vi "Add Async Methods Actor.vi"(8 "error in":errorcluster, 11 "Target Item":T1) -> (0 "error out":errorcluster)   [LabVIEW 2023, in "Add Async Methods Actor.lvlib"]
uses:
  Add Async Methods Actor.lvlib
  <resource>/Framework/Providers/API/mxLvNIIM.ctl
  Classes/Live Store/Live Store.lvclass
  Localized Strings.vi
  AFPP Shared/AFPP Shared.lvlib
  C:/Users/AndreaVaccaro(LSInst/Downloads/Projects/Async Methods Actor/Providers/AddAsyncMethodsActor/Classes/Actor Store/Actor Store.lvclass
  C:/Users/AndreaVaccaro(LSInst/Downloads/Projects/Async Methods Actor/Providers/AddAsyncMethodsActor/Classes/Live Store/Live Store.lvclass
panel:
  out "Path Display":string
  in  "Path":path caption="Save files to..."
  in  "Inherit from:":string(combo)
  in  "Cancel Button":bool
  in  "OK Button":bool
  in  "Name of Async Method Actor":string
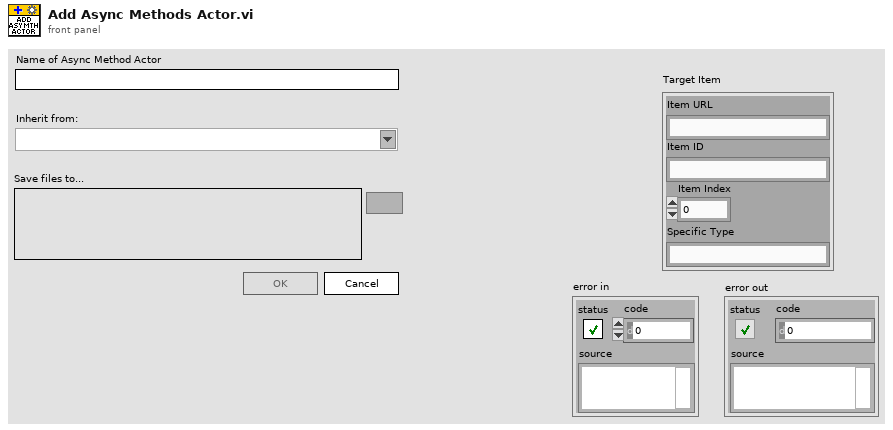
[diagram p1: front panel]
types:
  T1 = typedef "mxLvNIIM.ctl" = cluster{"Item URL":string, "Item ID":string, "Item Index":i32, "Specific Type":string}
  T2 = enum8{"Enabled", "Disabled", "Disabled and Grayed Out"}
  T3 = enum32{"Invalid", "Standard", "Closed", "Hidden", "Minimized", "Maximized"}
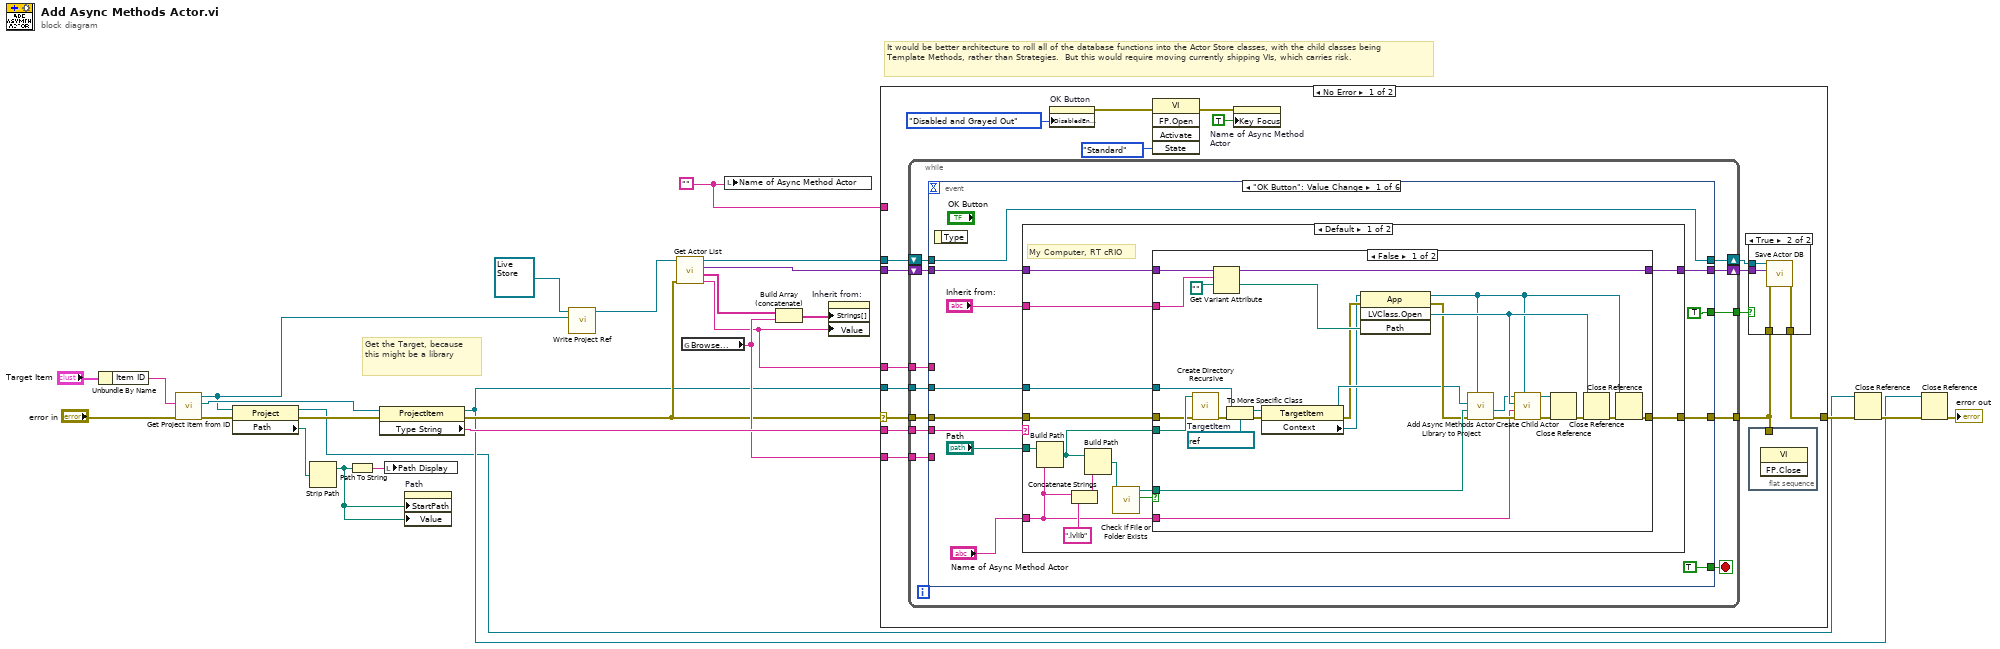
[diagram p0: block diagram]
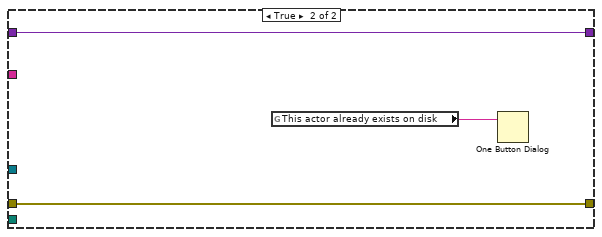
[diagram p2: hidden frame]
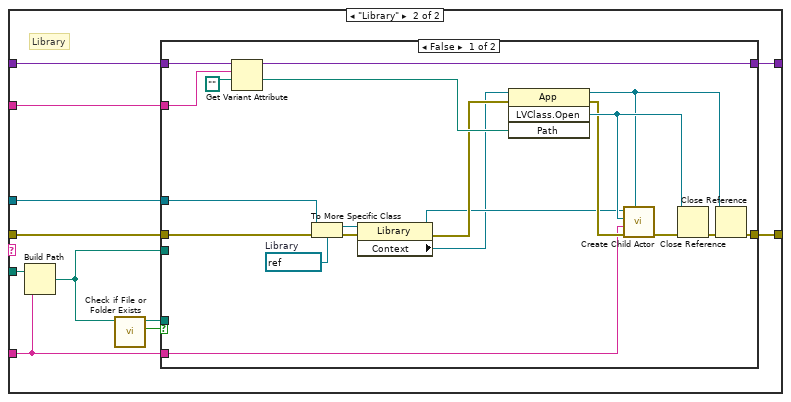
[diagram p3: hidden frame]
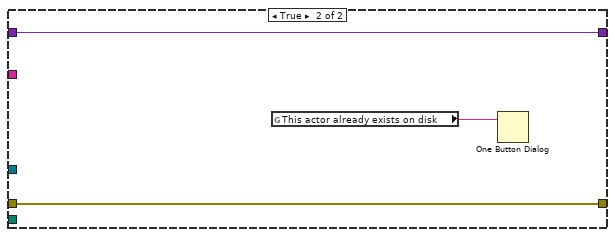
[diagram p4: hidden frame]
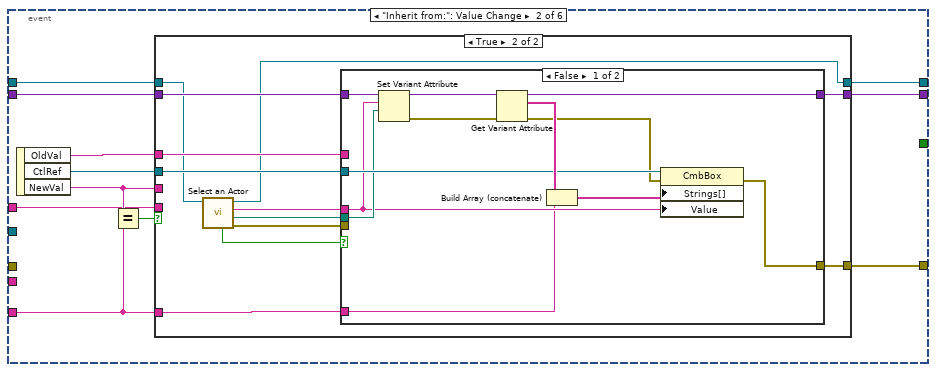
[diagram p5: hidden frame]
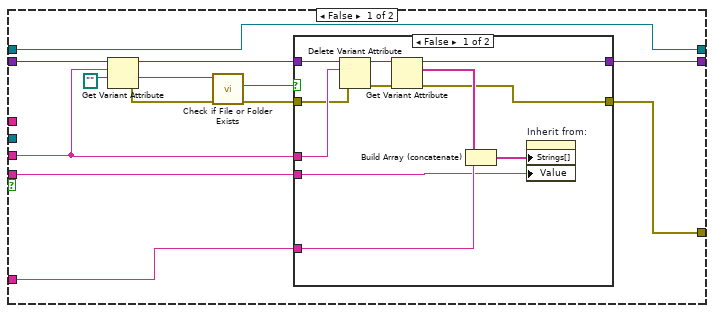
[diagram p6: hidden frame]
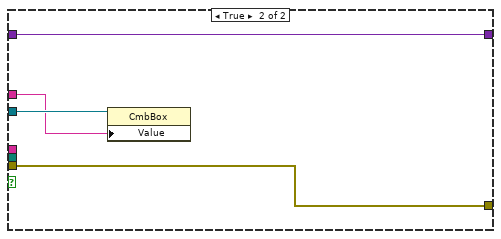
[diagram p8: hidden frame]
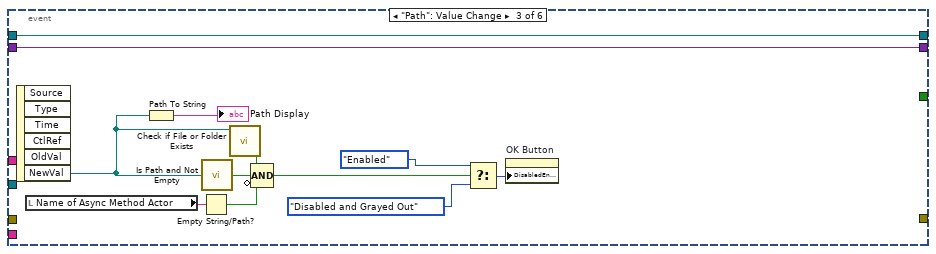
[diagram p9: hidden frame]
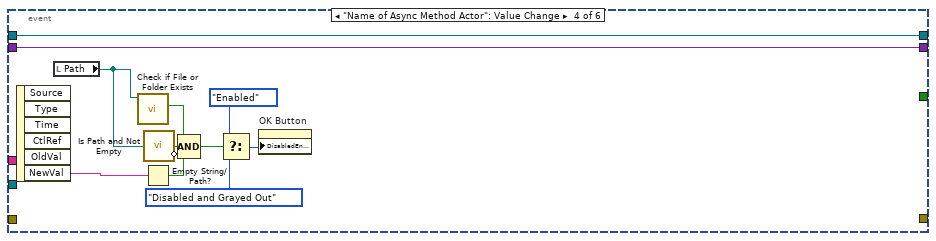
[diagram p10: hidden frame]
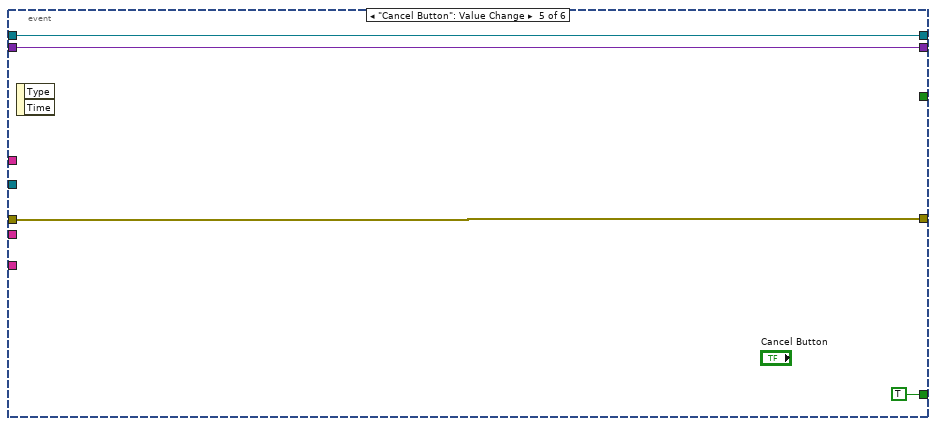
[diagram p11: hidden frame]
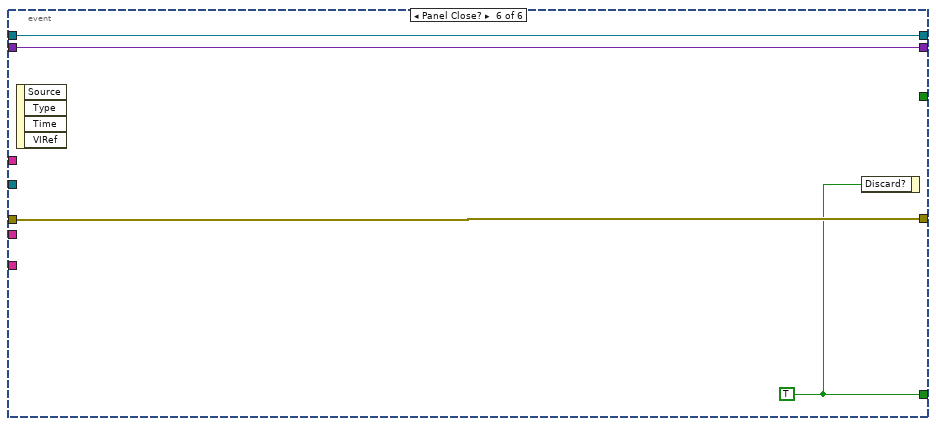
[diagram p12: hidden frame]
diagram:
  w10 = "" ("Name of Actor")
  # "Get the Target, because this might be a library"
  # "It would be better architecture to roll all of the database functions into the Actor Store classes, with the child classes being Template Methods, rather than Strategies.  But this would require moving currently shipping VIs, which carries risk."
  n1 = Unbundle By Name("Target Item") -> ("Item ID"=w7:string)
  n2 = call "Get Project Item from ID.vi"("error in (no error)"="error in", "Item ID"=w7) -> ("error out"=w4:errorcluster, "Project Item"=w3:refnum<vi>, "Project out"=w2:refnum<vi>)  [unwired: 7 in]
  n3 = property class="Project"(reference=w2, error in=w4) -> (reference out=w8:refnum<vi>, error out=w18:errorcluster, "Path"=w24:path)
  n4 = Strip Path(path=w24) -> (stripped path=w20:path)  [unwired: 1 out]
  n5 = Path To String(path=w20) -> (string=w21:string)
  n6 = property class="ProjectItem"(reference=w3, error in=w18) -> (reference out=w9:refnum<vi>, error out=w12:errorcluster, "Type String"=w23:string)
  n7 = local write "Path Display"(w21) -> ()
  n8 = property on="Path" class="Path"("StartPath"=w20, "Value"=w20) -> ()  [unwired: 2 in, 2 out]
  n9 = call-dynamic "Write Project Ref.vi"("Project Item"=w2, "Target Store in"=refnum<class "Live Store.lvclass"> refnum ("Add Async Methods Actor.lvlib:Live Store.lvclass")) -> ("Target Store out"=w17:refnum<class "Live Store.lvclass">)  [unwired: 9 in]
  n10 = call "Get Actor List.vi"("error in (no error)"=w12, "Actor Store"=w17) -> ("Actor Label"=w19:string, "Actors"=w15:string[], "Actor Paths"=w26:variant, "Actor Store"=w16:refnum<class "Live Store.lvclass">)  [unwired: 6 in]
  n11 = global read "Localized Strings.vi" "Browse..."() -> (w22:string)
  n12 = local write "Name of Async Method Actor"(w10) -> ()
  n13 = Build Array (concatenate)(w15, w22) -> (w25:string[])
  n14 = property on="Inherit from:" class="CmbBox"("Strings[]"=w25, "Value"=w19) -> ()  [unwired: 2 in, 2 out]
  n15 = case shown="No Error" w12 {
    selector: w12 -> [w43 w247]
    tunnel: [w37 w247] -> w13
    tunnel: w26 -> [w42 _]
    tunnel: w23 -> [w41 _]
    tunnel: w9 -> [w40 _]
    tunnel: w22 -> [w39 _]
    tunnel: w19 -> [w35 _]
    tunnel: w16 -> [w34 _]
    tunnel: w10 -> [_ _]
    frame No Error {
      n16 = while {
        tunnel: [w55] -> w31
        tunnel: w43 -> [w54]
        shift-right: [w51] -> w38
        shift-left: w42 -> [w52]
        tunnel: w41 -> [w50]
        tunnel: w40 -> [w49]
        tunnel: w39 -> [w48]
        tunnel: [w47] -> w36
        tunnel: w35 -> [w46]
        shift-right: [w44] -> w33
        shift-left: w34 -> [w45]
        stop <- w53 stop-if-true
        n17 = event shown="[0] \"OK Button\": Value Change" {
          selector: _ -> [_ _ _ _ _ _]
          dyn-events: _ -> [_ _ _ _ _ _]
          timeout: _ -> [_ _ _ _ _ _]
          tunnel: w54 -> [w61 _ _ _ w236 w241]
          tunnel: [w62 w156 _ _ w236 w241] -> w55
          tunnel: [TRUE _ _ _ TRUE w239] -> w53
          tunnel: w52 -> [w65 w155 w219 w226 w235 w240]
          tunnel: [w63 w154 w219 w226 w235 w240] -> w51
          tunnel: w50 -> [w60 _ _ _ _ _]
          tunnel: w49 -> [w59 _ _ _ _ _]
          tunnel: w48 -> [_ w150 _ _ _ _]
          tunnel: [TRUE _ _ _ _ _] -> w47
          tunnel: w46 -> [_ w149 _ _ _ _]
          tunnel: w45 -> [w56 w147 w211 w223 w234 w238]
          tunnel: [w56 w146 w211 w223 w234 w238] -> w44
          event "OK Button": Value Change {
            n18 = event-data() -> ()  [unwired: 1 in, 1 out]
            n19 = case shown="Default" w60 {
              tunnel: "Path" -> [w81 w122]
              tunnel: "Name of Async Method Actor" -> [w69 w113]
              tunnel: w65 -> [w80 w121]
              tunnel: "Inherit from:" -> [w79 w120]
              tunnel: [w78 w119] -> w63
              tunnel: [w75 w117] -> w62
              tunnel: w61 -> [w74 w116]
              tunnel: w59 -> [w72 w114]
              frame Default {
                # "My Computer, RT cRIO"
                n20 = Build Path(base path=w81, name or relative path=w69) -> (appended path=w77:path)
                n21 = Concatenate Strings(w69, ".lvlib" ("string")) -> (w70:string)
                n22 = Build Path(base path=w77, name or relative path=w70) -> (appended path=w68:path)
                n23 = call <vilib>:"Check if File or Folder Exists.vi"("path"=w68) -> ("file or folder exists?"=w73:bool, "dup path"=w76:path)  [unwired: 8 in, 1 out]
                n24 = case shown="False" w73 {
                  tunnel: w69 -> [w92 _]
                  tunnel: w80 -> [w107 w111]
                  tunnel: w79 -> [w106 _]
                  tunnel: [w105 w111] -> w78
                  tunnel: w77 -> [w91 _]
                  tunnel: w76 -> [w102 _]
                  tunnel: [w93 w110] -> w75
                  tunnel: w74 -> [w90 w110]
                  tunnel: w72 -> [w96 _]
                  frame False {
                    w101 = refnum<vi> refnum  # TargetItem
                    n25 = call <vilib>:"Create Directory Recursive.vi"("error in (no error)"=w90, "directory"=w91) -> ("error out"=w89:errorcluster)  [unwired: 3 in, 2 out]
                    n26 = Get Variant Attribute(Variant=w107, name=w106, default value (empty Variant)=path "") -> (duplicate Variant=w105:variant, value=w104:path)  [unwired: 1 in, 2 out]
                    n27 = To More Specific Class(target class=w101, reference=w96, error in=w89) -> (specific class reference=w88:refnum<vi>, error out=w86:errorcluster)
                    n28 = property class="TargetItem"(reference=w88, error in=w86) -> (reference out=w87:refnum<vi>, error out=w85:errorcluster, "Context"=w84:refnum<vi>)
                    n29 = invoke class="App" method="LVClass.Open"(reference=w84, error in=w85, "Path"=w104) -> (reference out=w83:refnum<vi>, error out=w95:errorcluster, "LVClass.Open"=w108:refnum<vi>)  [unwired: 1 in, 1 out]
                    n30 = call "Add Async Methods Actor Library to Project.vi"("Application"=w83, "error in (no error)"=w95, "Library Path"=w102, "Target Item"=w87) -> ("error out"=w100:errorcluster, "Library out"=w99:refnum<vi>)  [unwired: 6 in]
                    n31 = call "Create Child Actor.vi"("App Inst"=w83, "error in (no error)"=w100, "Actor Name"=w92, "Parent Class"=w108, "Library in"=w99) -> ("error out"=w98:errorcluster, "Library out"=w97:refnum<vi>)  [unwired: 5 in]
                    n32 = Close Reference(reference=w97, error in (no error)=w98) -> (error out=w82:errorcluster)
                    n33 = Close Reference(reference=w108, error in (no error)=w82) -> (error out=w94:errorcluster)
                    n34 = Close Reference(reference=w83, error in (no error)=w94) -> (error out=w93:errorcluster)
                  }
                  frame True {
                    n35 = global read "Localized Strings.vi" "This actor already exists on disk"() -> (w109:string)
                    n36 = One Button Dialog(message=w109) -> ()  [unwired: 1 in, 1 out]
                  }
                }
              }
              frame "Library" {
                # "Library"
                n37 = Build Path(base path=w122, name or relative path=w113) -> (appended path=w112:path)
                n38 = call <vilib>:"Check if File or Folder Exists.vi"("path"=w112) -> ("file or folder exists?"=w115:bool, "dup path"=w118:path)  [unwired: 8 in, 1 out]
                n39 = case shown="False" w115 {
                  tunnel: w113 -> [w131 _]
                  tunnel: w121 -> [w141 w145]
                  tunnel: w120 -> [w140 _]
                  tunnel: [w139 w145] -> w119
                  tunnel: w112 -> [_ _]
                  tunnel: w118 -> [_ _]
                  tunnel: [w132 w144] -> w117
                  tunnel: w116 -> [w130 w144]
                  tunnel: w114 -> [w135 _]
                  frame False {
                    w136 = refnum<vi> refnum  # Library
                    n40 = Get Variant Attribute(Variant=w141, name=w140, default value (empty Variant)=path "") -> (duplicate Variant=w139:variant, value=w138:path)  [unwired: 1 in, 2 out]
                    n41 = To More Specific Class(target class=w136, reference=w135, error in=w130) -> (specific class reference=w128:refnum<vi>, error out=w126:errorcluster)
                    n42 = property class="Library"(reference=w128, error in=w126) -> (reference out=w127:refnum<vi>, error out=w129:errorcluster, "Context"=w125:refnum<vi>)
                    n43 = invoke class="App" method="LVClass.Open"(reference=w125, error in=w129, "Path"=w138) -> (reference out=w124:refnum<vi>, error out=w134:errorcluster, "LVClass.Open"=w142:refnum<vi>)  [unwired: 1 in, 1 out]
                    n44 = call "Create Child Actor.vi"("App Inst"=w124, "error in (no error)"=w134, "Actor Name"=w131, "Parent Class"=w142, "Library in"=w127) -> ("error out"=w123:errorcluster)  [unwired: 5 in, 1 out]
                    n45 = Close Reference(reference=w142, error in (no error)=w123) -> (error out=w133:errorcluster)
                    n46 = Close Reference(reference=w124, error in (no error)=w133) -> (error out=w132:errorcluster)
                  }
                  frame True {
                    n47 = global read "Localized Strings.vi" "This actor already exists on disk"() -> (w143:string)
                    n48 = One Button Dialog(message=w143) -> ()  [unwired: 1 in, 1 out]
                  }
                }
              }
            }
          }
          event "Inherit from:": Value Change {
            n49 = event-data() -> ("OldVal"=w148:string, "CtlRef"=w153:refnum<vi>, "NewVal"=w151:string)  [unwired: 1 in]
            n50 = Equal?(x=w151, y=w150) -> (x = y?=w152:bool)
            n51 = case shown="True" w152 {
              tunnel: [w162 w188] -> w156
              tunnel: w155 -> [w169 w190]
              tunnel: [w163 w189] -> w154
              tunnel: w153 -> [_ w187]
              tunnel: w151 -> [w160 _]
              tunnel: w150 -> [w159 w186]
              tunnel: w149 -> [w158 _]
              tunnel: w148 -> [_ w185]
              tunnel: w147 -> [w157 w184]
              tunnel: [w157 w183] -> w146
              frame False {
                n52 = Get Variant Attribute(Variant=w169, name=w160, default value (empty Variant)=path "") -> (duplicate Variant=w166:variant, value=w168:path, error out=w165:errorcluster)  [unwired: 1 in, 1 out]
                n53 = call <vilib>:"Check if File or Folder Exists.vi"("error in (no error)"=w165, "path"=w168) -> ("error out"=w164:errorcluster, "file or folder exists?"=w161:bool)  [unwired: 7 in, 1 out]
                n54 = case shown="False" w161 {
                  tunnel: w166 -> [w180 w182]
                  tunnel: w160 -> [w179 _]
                  tunnel: w164 -> [w178 w181]
                  tunnel: [w173 w182] -> w163
                  tunnel: [w172 w181] -> w162
                  tunnel: w159 -> [w171 _]
                  tunnel: w158 -> [w170 _]
                  frame False {
                    n55 = Delete Variant Attribute(4:w178, 6:w179, 7:w180) -> (0:w174:errorcluster, 3:w177:variant)  [unwired: 1 out]
                    n56 = Get Variant Attribute(Variant=w177, error in=w174) -> (duplicate Variant=w173:variant, names=w175:string[], error out=w172:errorcluster)  [unwired: 2 in, 1 out]
                    n57 = Build Array (concatenate)(w175, w171) -> (w176:string[])
                    n58 = property on="Inherit from:" class="CmbBox"("Strings[]"=w176, "Value"=w170) -> ()  [unwired: 2 in, 2 out]
                  }
                  frame True {
                  }
                }
              }
              frame True {
                n59 = call "Select an Actor.vi"("Actor Store"=w184) -> ("error out"=w194:errorcluster, "Path to Actor"=w193:path, "Name of Actor"=w192:string, "Actor Store"=w183:refnum<class "Live Store.lvclass">, "Cancelled"=w191:bool)  [unwired: 6 in]
                n60 = case shown="False" w191 {
                  tunnel: w192 -> [w196 _]
                  tunnel: w193 -> [w198 _]
                  tunnel: w194 -> [_ w209]
                  tunnel: w190 -> [w200 w210]
                  tunnel: [w203 w210] -> w189
                  tunnel: [w201 w209] -> w188
                  tunnel: w187 -> [w205 w208]
                  tunnel: w186 -> [w195 _]
                  tunnel: w185 -> [_ w207]
                  frame False {
                    n61 = Set Variant Attribute(Variant=w200, name=w196, value=w198) -> (Variant out=w199:variant, error out=w197:errorcluster)  [unwired: 1 in, 1 out]
                    n62 = Get Variant Attribute(Variant=w199, error in=w197) -> (duplicate Variant=w203:variant, names=w206:string[], error out=w202:errorcluster)  [unwired: 2 in, 1 out]
                    n63 = Build Array (concatenate)(w206, w195) -> (w204:string[])
                    n64 = property class="CmbBox"(reference=w205, error in=w202, "Strings[]"=w204, "Value"=w196) -> (error out=w201:errorcluster)  [unwired: 1 out]
                  }
                  frame True {
                    n65 = property class="CmbBox"(reference=w208, "Value"=w207) -> ()  [unwired: 1 in, 2 out]
                  }
                }
              }
            }
          }
          event "Path": Value Change {
            n66 = event-data() -> ("NewVal"=w212:path)  [unwired: 1 in, 5 out]
            n67 = local read "Name of Async Method Actor"() -> (w218:string)
            n68 = Path To String(path=w212) -> (string=→"Path Display":string)
            n69 = Empty String/Path?(string/path=w218) -> (empty?=w217:bool)
            n70 = call <vilib>:"Is Path and Not Empty.vi"("path"=w212) -> ("Is Path and Not Empty?"=w216:bool)  [unwired: 4 in]
            n71 = call <vilib>:"Check if File or Folder Exists.vi"("path"=w212) -> ("file or folder exists?"=w213:bool)  [unwired: 8 in, 2 out]
            n72 = Compound Arithmetic op=AND(w213, w216, invert w217) -> (w215:bool)
            n73 = Select(t=T2."Enabled" ("Disabled"), s=w215, f=T2."Disabled and Grayed Out" ("Disabled")) -> (s? t:f=w221:T2)
            n74 = property on="OK Button" class="Bool"("DisabledEnum"=w221) -> ()  [unwired: 2 in, 2 out]
          }
          event "Name of Async Method Actor": Value Change {
            n75 = event-data() -> ("NewVal"=w227:string)  [unwired: 1 in, 5 out]
            n76 = local read "Path"() -> (w224:path)
            n77 = call <vilib>:"Check if File or Folder Exists.vi"("path"=w224) -> ("file or folder exists?"=w225:bool)  [unwired: 8 in, 2 out]
            n78 = Empty String/Path?(string/path=w227) -> (empty?=w230:bool)
            n79 = call <vilib>:"Is Path and Not Empty.vi"("path"=w224) -> ("Is Path and Not Empty?"=w229:bool)  [unwired: 4 in]
            n80 = Compound Arithmetic op=AND(w225, w229, invert w230) -> (w228:bool)
            n81 = Select(t=T2."Enabled" ("Disabled"), s=w228, f=T2."Disabled and Grayed Out" ("Disabled")) -> (s? t:f=w232:T2)
            n82 = property on="OK Button" class="Bool"("DisabledEnum"=w232) -> ()  [unwired: 2 in, 2 out]
          }
          event "Cancel Button": Value Change {
            n83 = event-data() -> ()  [unwired: 1 in, 2 out]
          }
          event Panel Close? {
            w239 = TRUE
            n84 = event-data() -> ()  [unwired: 1 in, 4 out]
            n85 = event-data("Discard?"=w239) -> ()  [unwired: 1 in, 1 out]
          }
        }
      }
      n86 = property on="OK Button" class="Bool"("DisabledEnum"=T2."Disabled and Grayed Out" ("Disabled")) -> (error out=w27:errorcluster)  [unwired: 2 in, 1 out]
      n87 = invoke class="VI" method="FP.Open"(error in=w27, "State"=T3."Standard") -> (error out=w29:errorcluster)  [unwired: 3 in, 4 out]
      n88 = property on="Name of Async Method Actor" class="Str"(error in=w29, "Key Focus"=TRUE) -> ()  [unwired: 1 in, 2 out]
      n89 = case shown="True" w36 {
        tunnel: w38 -> [_ w244]
        tunnel: [w242 w246] -> w37
        tunnel: w31 -> [w242 w245]
        tunnel: w33 -> [_ w243]
        frame False {
        }
        frame True {
          n90 = call "Save Actor DB.vi"("error in (no error)"=w245, "Actor DB"=w244, "Actor Store"=w243) -> ("error out"=w246:errorcluster)  [unwired: 6 in, 2 out]
        }
      }
      n91 = flat-sequence {
        tunnel: w31 -> [_]
        frame #0 {
          n92 = invoke class="VI" method="FP.Close"() -> ()  [unwired: 3 in, 3 out]
        }
      }
    }
    frame Error {
    }
  }
  n93 = Close Reference(reference=w8, error in (no error)=w13) -> (error out=w14:errorcluster)
  n94 = Close Reference(reference=w9, error in (no error)=w14) -> (error out=→"error out":errorcluster)
